vi "Delete Old Log Files.vi"(8 "error in (no error)":errorcluster, 11 "Error Handler In":refnum<class "Error Handler.lvclass">) -> (0 "error out":errorcluster, 3 "Error Handler Out":refnum<class "Error Handler.lvclass">)   [LabVIEW 2020, in "Error Handler.lvclass"]
uses:
  Error Handler.lvclass
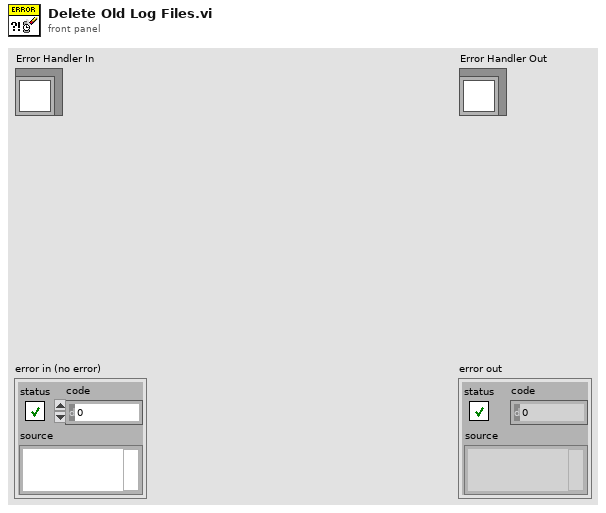
[diagram p1: front panel]
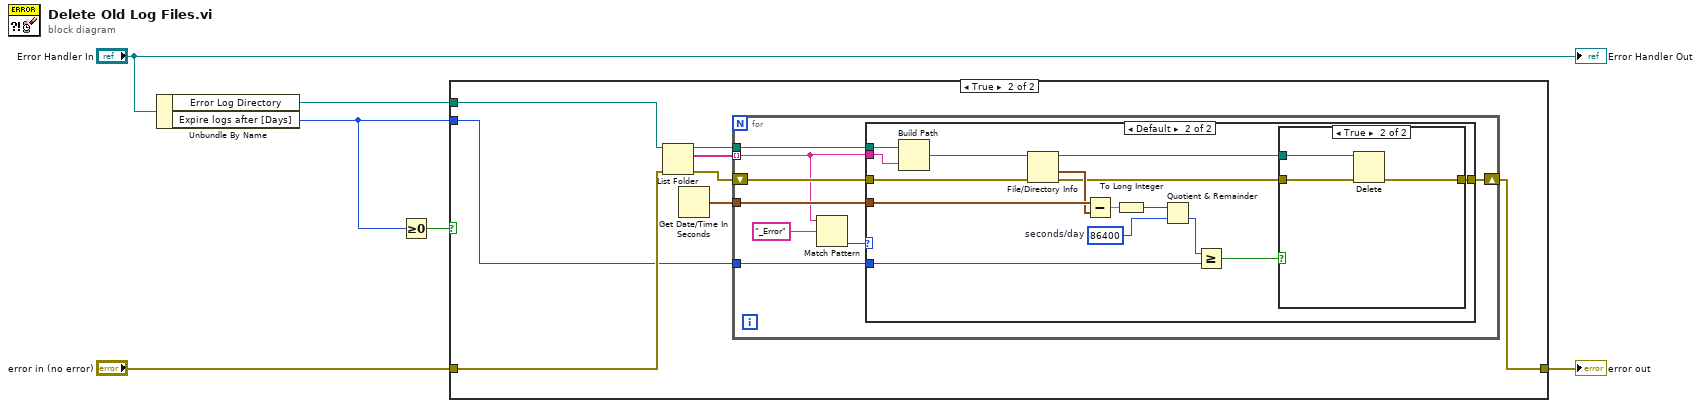
[diagram p0: block diagram]
diagram:
  n1 = Unbundle By Name("Error Handler In") -> ("Error Log Directory"=w2:path, "Expire logs after [Days]"=w1:i32)
  n2 = Greater Or Equal To 0?(x=w1) -> (x >= 0?=w3:bool)
  n3 = case shown="True" w3 {
    tunnel: [w7 w11] -> w6
    tunnel: "error in (no error)" -> [w7 w10]
    tunnel: w1 -> [_ w9]
    tunnel: w2 -> [_ w8]
    frame False {
      # "Expiration time less than 0 -> never expire."
    }
    frame True {
      n4 = List Folder(path=w8, error in=w10) -> (path out=w14:path, filenames=w15:string[], error out=w13:errorcluster)  [unwired: 2 in, 1 out]
      n5 = Get Date/Time In Seconds() -> (seconds since 1Jan1904=w12:timestamp)
      n6 = for {
        tunnel: w15 -> [w18] mode=indexing
        tunnel: w14 -> [w23]
        shift-right: [w20] -> w11
        shift-left: w13 -> [w19]
        tunnel: w12 -> [w22]
        tunnel: w9 -> [w21]
        n7 = Match Pattern(string=w18, regular expression="_Error") -> (offset past match=w16:i32)  [unwired: 1 in, 3 out]
        n8 = case shown="Default" w16 {
          tunnel: w23 -> [_ w39]
          tunnel: w22 -> [_ w37]
          tunnel: w21 -> [_ w31]
          tunnel: [w24 w27] -> w20
          tunnel: w19 -> [w24 w26]
          tunnel: w18 -> [_ w25]
          frame -1 {
          }
          frame Default {
            w34 = 86400  # seconds/day
            n9 = Build Path(base path=w39, name or relative path=w25) -> (appended path=w38:path)
            n10 = File/Directory Info(path=w38, error in=w26) -> (path out=w28:path, last mod=w36:timestamp, error out=w29:errorcluster)  [unwired: 4 out]
            n11 = Subtract(x=w37, y=w36) -> (x-y=w35:dbl)
            n12 = To Long Integer(number=w35) -> (32bit integer=w33:i32)
            n13 = Quotient & Remainder(x=w33, y=w34) -> (floor(x/y)=w32:i32)  [unwired: 1 out]
            n14 = Greater Or Equal?(x=w32, y=w31) -> (x >= y?=w30:bool)
            n15 = case shown="True" w30 {
              tunnel: w29 -> [w40 w42]
              tunnel: w28 -> [_ w43]
              tunnel: [w40 w41] -> w27
              frame False {
              }
              frame True {
                n16 = Delete(path (use dialog)=w43, error in=w42) -> (error out=w41:errorcluster)  [unwired: 3 in, 2 out]
              }
            }
          }
        }
      }
    }
  }
  "error out" <- w6
  "Error Handler Out" <- "Error Handler In"
